vi "Packet1+Packet2.vi"() -> ()   [LabVIEW 2012]
uses:
  <vilib>/addons/Modulation/Digital/General/MT Generate PSK System Parameters(M).vi
  <instrlib>/niUSRP/niUSRP Write Tx Data (CDB Cluster).vi
  <vilib>/addons/Modulation/niDMT.lvlib
panel:
  out "Numeric 2":i32
  in  "Stop the \nTransmission":bool
  out "millisecond timer value 3":u32
  out "Numeric":u32
  out "output cluster":T1
  in  "Referance Cluster":T1={"Tx IQ Sampling\nRate [s/sec]"=500000.0, "Tx Frequency [Hz]"=2500000000.0, "Tx Gain [dB]"=0.0, "Tx Antenna"="TX1"} {"Tx Gain [dB]" format="%#.6p"; "Tx Frequency [Hz]" format="%#.6p"; "Tx IQ Sampling\nRate [s/sec]" format="%#.6p"}
  out "Transmission\n       Stop":bool
  in  "end of data?":bool
  out "Constellation Graph 2":T2(graph) caption="Constellation Graph"
  in  "autoscale 2":bool caption="autoscale"
  out "error out 3":errorcluster
  in  "Tab Control 2":T3(tab)
  in  "Transmitted Message":string
  out "M-ary":i32
  in  "Packet Parameters 2":T4={"Guard Bits "=30, "Sync Bits"=20, "Message Bits"=128}
  in  "Packet Pad \n[samples] 2":i32=200
  in  "Blank Frame \n[samples] 2":i32=500
  out "Number of Packets in Message 2":i32=46
  in  "PN sequence order\nfor Sync Bits 2":i32=31 caption="PN sequence order (9)"
  in  "Packet Repeat 2":i32=2
  in  "Pulse Shaping Filter Parameters 2":T5={"Alpha"=0.5, "Filter Length"=6, "TX Filter"=enum."Root Raised Cos"} caption="Pulse Shaping Filter" {"Alpha" format="%.2f"}
  out "Actual Tx Parameters 2":T1={"Tx IQ Sampling\nRate [s/sec]"=200000.0, "Tx Frequency [Hz]"=2500000000.0, "Tx Gain [dB]"=0.0, "Tx Antenna"="TX1"} {"Tx Gain [dB]" format="%#.6p"; "Tx Frequency [Hz]" format="%#.6p"; "Tx IQ Sampling\nRate [s/sec]" format="%#.6p"}
  out "error out 2":errorcluster
  in  "Queue Length 2":i32=10
  in  "BPSK System Parameters 9":T6={"Samples per Symbol"=8, "symbol map"=[], "Differential PSK"=enum."disable", "PSK type"=0} caption="BPSK System Parameters" {"PSK type" items=["normal", "shifted", "offset"]; "symbol map" format="%.3f"}
  in  "BPSK System Parameters 8":T6={"Samples per Symbol"=8, "symbol map"=[], "Differential PSK"=enum."disable", "PSK type"=0} caption="BPSK System Parameters" {"PSK type" items=["normal", "shifted", "offset"]; "symbol map" format="%.3f"}
  in  "BPSK System Parameters 7":T6={"Samples per Symbol"=8, "symbol map"=[], "Differential PSK"=enum."disable", "PSK type"=0} caption="BPSK System Parameters" {"PSK type" items=["normal", "shifted", "offset"]; "symbol map" format="%.3f"}
  in  "BPSK System Parameters 6":T6={"Samples per Symbol"=8, "symbol map"=[], "Differential PSK"=enum."disable", "PSK type"=0} caption="BPSK System Parameters" {"PSK type" items=["normal", "shifted", "offset"]; "symbol map" format="%.3f"}
  in  "BPSK System Parameters 5":T6={"Samples per Symbol"=8, "symbol map"=[], "Differential PSK"=enum."disable", "PSK type"=0} caption="BPSK System Parameters" {"PSK type" items=["normal", "shifted", "offset"]; "symbol map" format="%.3f"}
  in  "BPSK System Parameters 4":T6={"Samples per Symbol"=8, "symbol map"=[], "Differential PSK"=enum."disable", "PSK type"=0} caption="BPSK System Parameters" {"PSK type" items=["normal", "shifted", "offset"]; "symbol map" format="%.3f"}
  in  "BPSK System Parameters 3":T6={"Samples per Symbol"=8, "symbol map"=[], "Differential PSK"=enum."disable", "PSK type"=0} caption="BPSK System Parameters" {"PSK type" items=["normal", "shifted", "offset"]; "symbol map" format="%.3f"}
  out "Symbol Rate\n[symbols/sec] 2":dbl=25000.0 format="%#.6p"
  out "millisecond timer value":u32
  in  "Tab Control":T3(tab)
  in  "Enter Control Signal\n         (1,2 or 3)":string
  out "The Transmission of \nControl Signal is stopped":bool
  out "Constellation Graph":T2(graph)
  out "Required \nPower Gain":dbl
  in  "Packet Parameters":T4={"Guard Bits "=30, "Sync Bits"=20, "Message Bits"=128}
  in  "Packet Pad \n[samples]":i32=200
  in  "Blank Frame \n[samples]":i32=500
  out "Number of Packets in Message":i32=46
  in  "PN sequence order\nfor Sync Bits":i32=31 caption="PN sequence order (9)"
  in  "Packet Repeat":i32=2
  in  "Select PSK Modulation Format":T7(tab)=enum."QPSK" caption="PSK"
  in  "BPSK System Parameters":T6={"Samples per Symbol"=8, "symbol map"=[], "Differential PSK"=enum."disable", "PSK type"=0} {"PSK type" items=["normal", "shifted", "offset"]; "symbol map" format="%.3f"}
  in  "QPSK System Parameters":T6={"Samples per Symbol"=8, "symbol map"=[], "Differential PSK"=enum."disable", "PSK type"=0} {"PSK type" items=["normal", "shifted", "offset"]; "symbol map" format="%.3f"}
  in  "pi/4 DQPSK System Parameters":T6={"Samples per Symbol"=8, "symbol map"=[], "Differential PSK"=enum."enable", "PSK type"=1} {"PSK type" items=["normal", "shifted", "offset"]; "symbol map" format="%.3f"}
  in  "OQPSK System Parameters":T6={"Samples per Symbol"=8, "symbol map"=[], "Differential PSK"=enum."disable", "PSK type"=2} {"PSK type" items=["normal", "shifted", "offset"]; "symbol map" format="%.3f"}
  in  "8-PSK System Parameters":T6={"Samples per Symbol"=8, "symbol map"=[], "Differential PSK"=enum."disable", "PSK type"=0} {"PSK type" items=["normal", "shifted", "offset"]; "symbol map" format="%.3f"}
  in  "16-PSK System Parameters":T6={"Samples per Symbol"=8, "symbol map"=[], "Differential PSK"=enum."disable", "PSK type"=0} {"PSK type" items=["normal", "shifted", "offset"]; "symbol map" format="%.3f"}
  in  "M":i32=4 min=2 step=2
  in  "Custom System Parameters":T6={"Samples per Symbol"=8, "symbol map"=[], "Differential PSK"=enum."disable", "PSK type"=0} {"PSK type" items=["normal", "shifted", "offset"]; "symbol map" format="%.3f"}
  in  "Pulse Shaping Filter Parameters":T5={"Alpha"=0.5, "Filter Length"=6, "TX Filter"=enum."Root Raised Cos"} caption="Pulse Shaping Filter" {"Alpha" format="%.2f"}
  in  "Tx Parameters":T1={"Tx IQ Sampling\nRate [s/sec]"=500000.0, "Tx Frequency [Hz]"=2500000000.0, "Tx Gain [dB]"=0.0, "Tx Antenna"="TX1"} {"Tx Gain [dB]" format="%#.6p"; "Tx Frequency [Hz]" format="%#.6p"; "Tx IQ Sampling\nRate [s/sec]" format="%#.6p"}
  out "Actual Tx Parameters":T1={"Tx IQ Sampling\nRate [s/sec]"=200000.0, "Tx Frequency [Hz]"=2500000000.0, "Tx Gain [dB]"=0.0, "Tx Antenna"="TX1"} {"Tx Gain [dB]" format="%#.6p"; "Tx Frequency [Hz]" format="%#.6p"; "Tx IQ Sampling\nRate [s/sec]" format="%#.6p"}
  in  "USRP IP address":refnum<k15>="192.168.10.2"
  out "error out":errorcluster
  in  "Queue Length":i32=10
  in  "autoscale":bool
  out "Symbol Rate\n[symbols/sec]":dbl=25000.0 format="%#.6p"
  in  "stop":bool
  # "Guard\nBand"
  # "Sync\nSeq"
  # "Packet\nNumber"
  # "Pad\nData"
  # "Blank\nFrame"
  # "Data"
  # "Guard\nBand"
  # "Sync\nSeq"
  # "Packet\nNumber"
  # "Pad\nData"
  # "Blank\nFrame"
  # "Data"
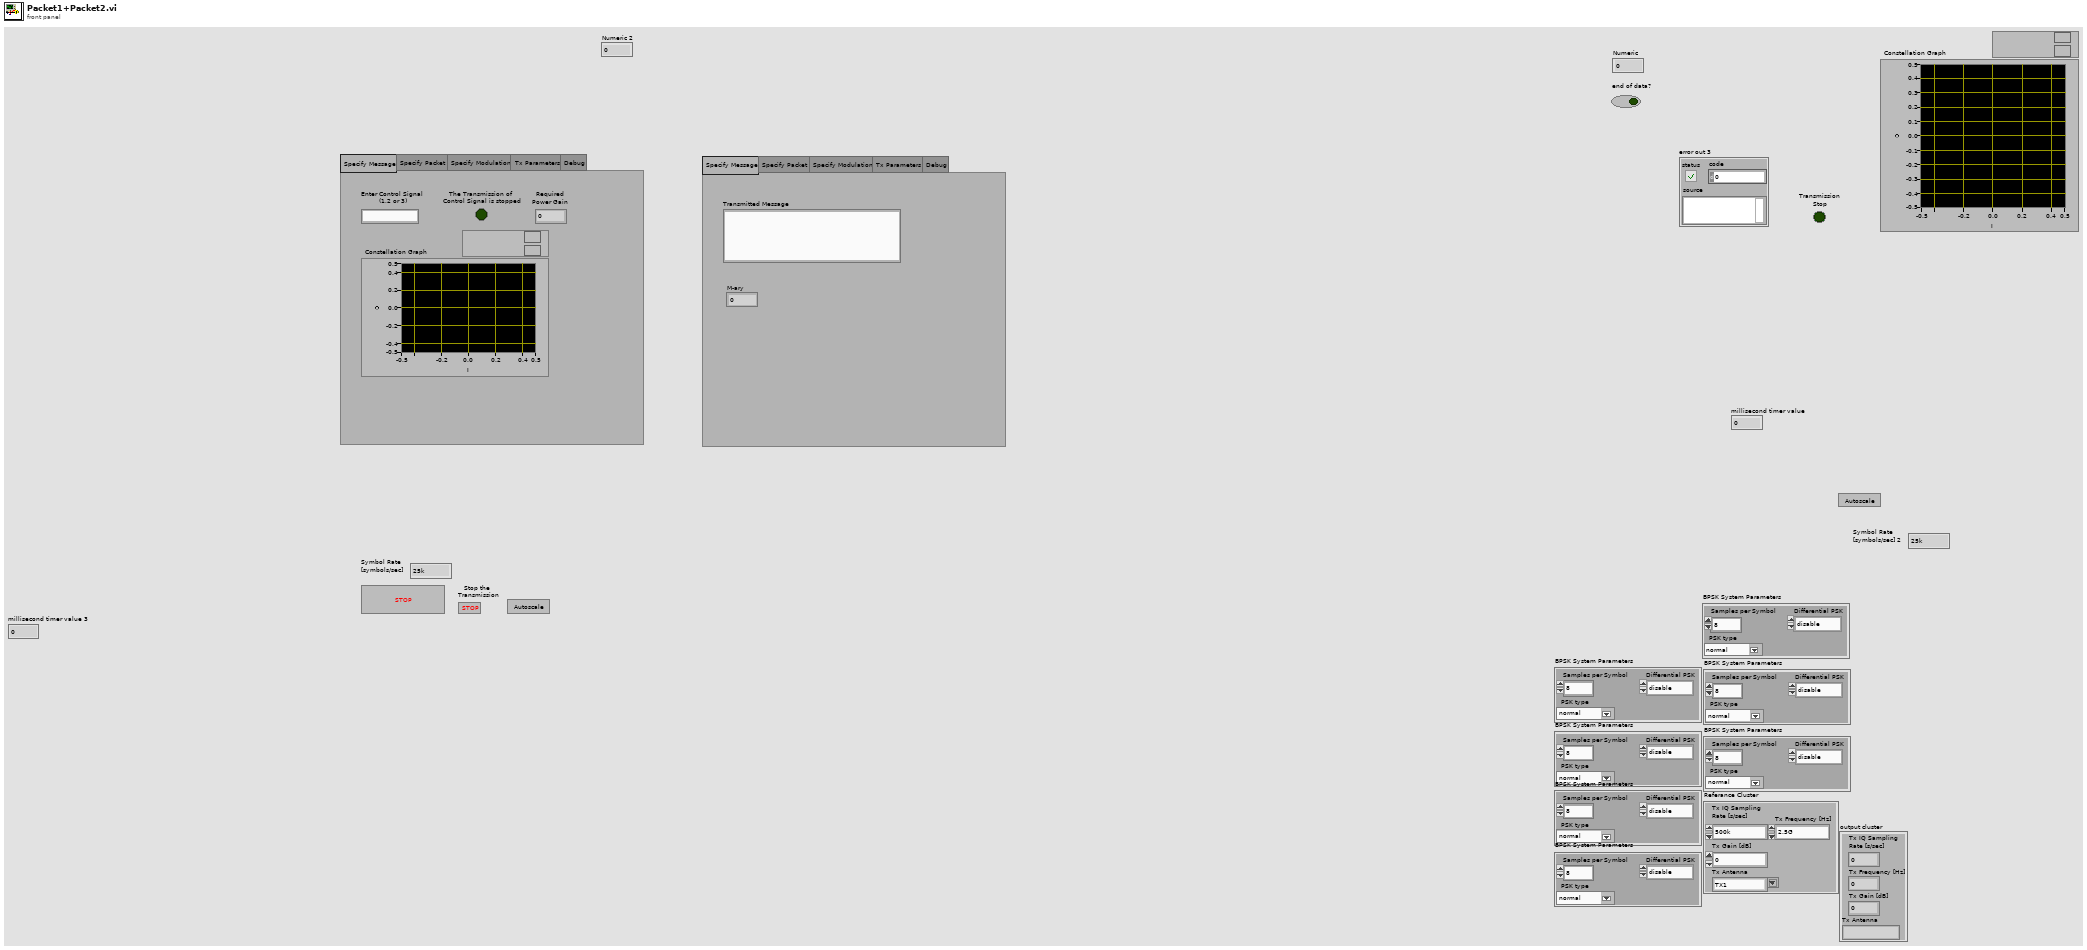
[diagram p1: front panel]
types:
  T1 = cluster{"Tx IQ Sampling\nRate [s/sec]":dbl, "Tx Frequency [Hz]":dbl, "Tx Gain [dB]":dbl, "Tx Antenna":string}
  T2 = cluster{"Decimated Array":dbl[], "Decimated Array":dbl[]}[]
  T3 = enum32{"Specify Message", "Specify Packet", "Specify Modulation", "Tx Parameters", "Debug"}
  T4 = cluster{"Guard Bits ":i32, "Sync Bits":i32, "Message Bits":i32}
  T5 = cluster{"Alpha":dbl, "Filter Length":i32, "TX Filter":enum16{"none", "Raised Cosine", "Root Raised Cos", "Gaussian"}}
  T6 = cluster{"Samples per Symbol":i32, "symbol map":cdb[], "Differential PSK":enum16{"disable", "enable"}, "PSK type":u16}
  T7 = enum32{"BPSK", "QPSK", "pi/4DQPSK", "OQPSK", "8-PSK", "16-PSK", "Custom"}
  T8 = cluster{"samples per symbol (16)":i32, "symbol map":cdb[], "differential PSK":enum16{"disable", "enable"}, "PSK type":u16}
  T9 = cluster{"s? t:f":cluster{"t0":dbl, "dt":dbl, "Y":cdb[]}, i32}
  T10 = cluster{"output complex waveform":cluster{"t0":dbl, "dt":dbl, "Y":cdb[]}, i32}
  T11 = cluster{"constellation":dbl[], "oversampled data":dbl[]}[]
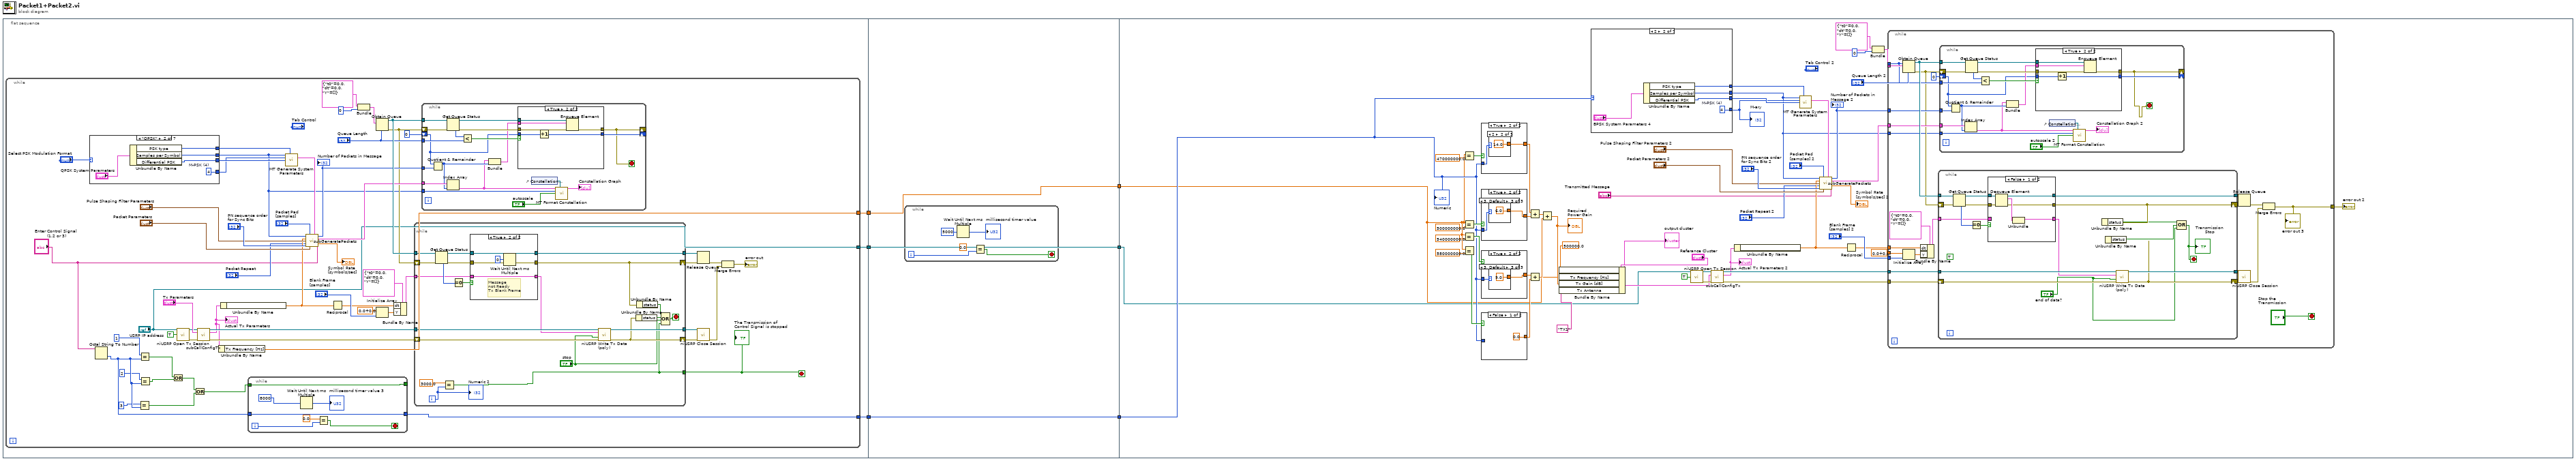
[diagram p0: block diagram]
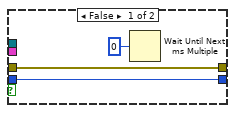
[diagram p2: hidden frame]
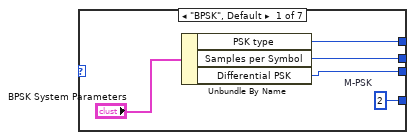
[diagram p3: hidden frame]
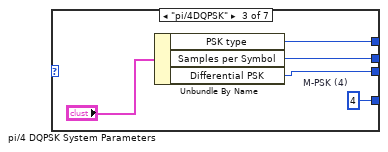
[diagram p4: hidden frame]
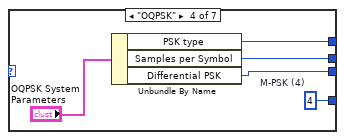
[diagram p5: hidden frame]
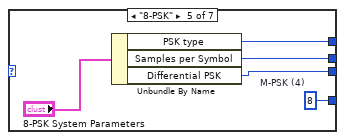
[diagram p6: hidden frame]
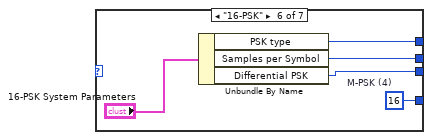
[diagram p7: hidden frame]
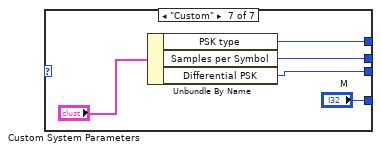
[diagram p8: hidden frame]
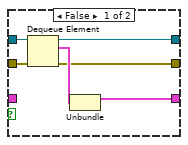
[diagram p9: hidden frame]
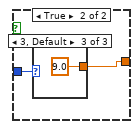
[diagram p10: hidden frame]
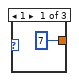
[diagram p11: hidden frame]
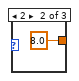
[diagram p12: hidden frame]
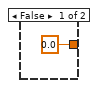
[diagram p13: hidden frame]
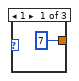
[diagram p14: hidden frame]
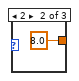
[diagram p15: hidden frame]
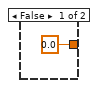
[diagram p16: hidden frame]
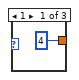
[diagram p17: hidden frame]
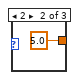
[diagram p18: hidden frame]
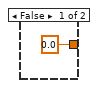
[diagram p19: hidden frame]
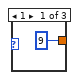
[diagram p20: hidden frame]
diagram:
  n1 = flat-sequence {
    tunnel: [w9] -> w5
    tunnel: [w8] -> w3
    tunnel: [w7] -> w1
    tunnel: [w169] -> w6
    tunnel: w5 -> [w169]
    tunnel: [w168] -> w4
    tunnel: w3 -> [w168]
    tunnel: [w167] -> w2
    tunnel: w1 -> [w167]
    tunnel: w6 -> [w177]
    tunnel: w4 -> [w176]
    tunnel: w2 -> [w175]
    frame #0 {
      n2 = while {
        tunnel: [w15] -> w9
        tunnel: [w13] -> w8
        tunnel: ["USRP IP address"] -> w7
        stop <- w11 stop-if-true
        n3 = case shown="\"QPSK\"" "Select PSK Modulation Format" {
          tunnel: [w102 w106 w114 w119 w124 w130 w133] -> w27
          tunnel: [w103 w108 w113 w118 w123 w129 w134] -> w64
          tunnel: [w105 w110 w115 w120 w122 w128 "M"] -> w46
          tunnel: [w104 w109 w112 w117 w125 w127 w135] -> w35
          frame "BPSK", Default {
            w105 = 2  # M-PSK
            n4 = Unbundle By Name("BPSK System Parameters") -> ("PSK type"=w104:u16, "Samples per Symbol"=w102:i32, "Differential PSK"=w103:enum16{"disable", "enable"})
          }
          frame "QPSK" {
            w110 = 4  # M-PSK (4)
            n5 = Unbundle By Name("QPSK System Parameters") -> ("PSK type"=w109:u16, "Samples per Symbol"=w106:i32, "Differential PSK"=w108:enum16{"disable", "enable"})
          }
          frame "pi/4DQPSK" {
            w115 = 4  # M-PSK (4)
            n6 = Unbundle By Name("pi/4 DQPSK System Parameters") -> ("PSK type"=w112:u16, "Samples per Symbol"=w114:i32, "Differential PSK"=w113:enum16{"disable", "enable"})
          }
          frame "OQPSK" {
            w120 = 4  # M-PSK (4)
            n7 = Unbundle By Name("OQPSK System Parameters") -> ("PSK type"=w117:u16, "Samples per Symbol"=w119:i32, "Differential PSK"=w118:enum16{"disable", "enable"})
          }
          frame "8-PSK" {
            w122 = 8  # M-PSK (4)
            n8 = Unbundle By Name("8-PSK System Parameters") -> ("PSK type"=w125:u16, "Samples per Symbol"=w124:i32, "Differential PSK"=w123:enum16{"disable", "enable"})
          }
          frame "16-PSK" {
            w128 = 16  # M-PSK (4)
            n9 = Unbundle By Name("16-PSK System Parameters") -> ("PSK type"=w127:u16, "Samples per Symbol"=w130:i32, "Differential PSK"=w129:enum16{"disable", "enable"})
          }
          frame "Custom" {
            n10 = Unbundle By Name("Custom System Parameters") -> ("PSK type"=w135:u16, "Samples per Symbol"=w133:i32, "Differential PSK"=w134:enum16{"disable", "enable"})
          }
        }
        n11 = Octal String To Number(4:"Enter Control Signal\n         (1,2 or 3)") -> (0:w19:u32)  [unwired: 2 in, 1 out]
        n12 = Equal?(x=3, y=w19) -> (x = y?=w21:bool)
        n13 = Equal?(x=1, y=w19) -> (x = y?=w24:bool)
        n14 = Equal?(x=2, y=w19) -> (x = y?=w23:bool)
        n15 = Or(x=w24, y=w23) -> (x .or. y?=w22:bool)
        n16 = call <instrlib>:"niUSRP Open Tx Session.vi"("device names"="USRP IP address", "reset"=TRUE) -> ("session handle out"=w38:refnum<k15>, "error out"=w37:errorcluster)  [unwired: 12 in]
        n17 = Or(x=w22, y=w21) -> (x .or. y?=w20:bool)
        n18 = call "subCallConfigTx.vi"("session handle"=w38, "Tx Parameters"="Tx Parameters", "error in"=w37) -> ("session handle out"=w45:refnum<k15>, "Actual Tx Parameters"=w14:T1, "error out"=w50:errorcluster)  [unwired: 10 in]
        "Actual Tx Parameters" <- w14
        n19 = Unbundle By Name(w14) -> ("Tx Frequency [Hz]"=w13:dbl)
        n20 = Unbundle By Name(w14) -> ("Tx IQ Sampling\nRate [s/sec]"=w28:dbl)
        n21 = while {
          tunnel: w20 -> [w71]
          tunnel: [w71] -> _
          tunnel: w19 -> [w70]
          tunnel: [w70] -> w15
          i -> [w68]
          stop <- w67 stop-if-true
          n22 = Wait Until Next ms Multiple(millisecond multiple=u32 8000) -> (millisecond timer value=→"millisecond timer value 3":u32)
          n23 = Equal?(x=0.0, y=w68) -> (x = y?=w67:bool)
        }
        n24 = call-poly <vilib>:"MT Generate System Parameters.vi"("samples per symbol (16)"=w27, "PSK type"=w35, "M-PSK (4)"=w46, "differential PSK"=w64) -> ("PSK system parameters"=w36:T8)  [unwired: 9 in, 2 out]
        n25 = call "subGeneratePackets.vi"("Samples per Symbol"=w27, "Packet Pad \n[samples]"="Packet Pad \n[samples]", "PSK system parameters"=w36, "Tx IQ Sampling\nRate [s/sec]"=w28, "Pulse Shaping Filter Parameters"="Pulse Shaping Filter Parameters", "Packet Repeat"="Packet Repeat", "PN sequence order\nfor Sync Bits"="PN sequence order\nfor Sync Bits", "Packet Parameters"="Packet Parameters", "Message Text"="Enter Control Signal\n         (1,2 or 3)") -> ("Number of Packets"=w44:i32, "Packets"=w52:cluster{"t0":dbl, "dt":dbl, "Y":cdb[]}[], "Symbol Rate"=→"Symbol Rate\n[symbols/sec]":dbl)  [unwired: 4 in]
        "Number of Packets in Message" <- w44
        n26 = Reciprocal(x=w28) -> (1/x=w47:dbl)
        n27 = Bundle("s? t:f"=cluster{"t0":dbl, "dt":dbl, "Y":cdb[]} {"t0"=0.0, "dt"=0.0, "Y"=[]}, 0) -> (w55:T9)  [unwired: 1 in]
        n28 = Obtain Queue(max queue size (-1, unlimited)="Queue Length", element data type=w55) -> (queue out=w61:refnum<queue>, error out=w40:errorcluster)  [unwired: 3 in, 1 out]
        n29 = Initialize Array(cdb 0.0+0.0i ("element"), "Blank Frame \n[samples]") -> (w60:cdb[])
        n30 = Bundle By Name(cluster=cluster{"t0":dbl, "dt":dbl, "Y":cdb[]} {"t0"=0.0, "dt"=0.0, "Y"=[]} ("s? t:f"), "dt"=w47, "Y"=w60) -> (w59:cluster{"t0":dbl, "dt":dbl, "Y":cdb[]})
        n31 = while {
          tunnel: w45 -> [w147]
          shift-right: [w144] -> w49
          shift-left: w50 -> [w148]
          tunnel: w61 -> [w156]
          tunnel: w59 -> [w153]
          tunnel: [w152] -> w58
          tunnel: [w146] -> w48
          shift-right: [w141] -> w57
          shift-left: w40 -> [w149]
          tunnel: [w136] -> w11
          i -> [w137]
          stop <- w143 stop-if-true
          n32 = Get Queue Status(queue=w156, error in (no error)=w149) -> (queue out=w151:refnum<queue>, error out=w150:errorcluster, # elements in queue=w155:i32)  [unwired: 1 in, 5 out]
          n33 = Equal?(x=3000.0, y=w137) -> (x = y?=w136:bool)
          n34 = Equal To 0?(x=w155) -> (x = 0?=w154:bool)
          n35 = case shown="True" w154 {
            tunnel: w153 -> [_ w166]
            tunnel: [w158 w166] -> w139
            tunnel: [w162 w164] -> w152
            tunnel: [w157 w165] -> w141
            tunnel: w151 -> [w161 w164]
            tunnel: w150 -> [w160 w165]
            frame False {
              n36 = Dequeue Element(queue=w161, error in (no error)=w160) -> (queue out=w162:refnum<queue>, element=w159:T9, error out=w157:errorcluster)  [unwired: 1 in, 1 out]
              n37 = Unbundle(w159) -> ("s? t:f"=w158:cluster{"t0":dbl, "dt":dbl, "Y":cdb[]})  [unwired: 1 out]
            }
            frame True {
              # "Message\nnot Ready\nTx Blank Frame"
              n38 = Wait Until Next ms Multiple(millisecond multiple=u32 0) -> ()  [unwired: 1 out]
            }
          }
          n39 = call-poly <instrlib>:"niUSRP Write Tx Data (poly).vi"("session handle"=w147, "data"=w139, "end of data?"="stop", "error in (no error)"=w148) -> ("session handle out"=w146:refnum<k15>, "error out"=w144:errorcluster)  [unwired: 10 in]
          n40 = Unbundle By Name(w144) -> ("status"=w145:bool)
          n41 = Unbundle By Name(w141) -> ("status"=w140:bool)
          n42 = Compound Arithmetic op=OR(w140, w145, "stop", w136) -> (w143:bool)
          "Numeric 2" <- w137
        }
        "The Transmission of \nControl Signal is stopped" <- w11
        n43 = while {
          tunnel: w61 -> [w91]
          shift-right: [w84] -> _
          shift-left: 0 -> [w80]
          tunnel: w52 -> [w81]
          tunnel: "Queue Length" -> [w83]
          tunnel: w44 -> [w82]
          shift-right: [w78] -> _
          shift-left: w40 -> [w86]
          tunnel: w27 -> [w75]
          stop <- w78 stop-if-true
          n44 = Quotient & Remainder(x=w80, y=w82) -> (x-y*floor(x/y)=w79:i32)  [unwired: 1 out]
          n45 = Index Array(array=w81, index=w79) -> (element=w73:cluster{"t0":dbl, "dt":dbl, "Y":cdb[]})
          n46 = Get Queue Status(queue=w91, error in (no error)=w86) -> (queue out=w90:refnum<queue>, error out=w87:errorcluster, # elements in queue=w89:i32)  [unwired: 1 in, 5 out]
          n47 = Less?(x=w89, y=w83) -> (x < y?=w88:bool)
          n48 = Bundle("output complex waveform"=w73, w79) -> (w85:T10)  [unwired: 1 in]
          n49 = case shown="True" w88 {
            tunnel: w87 -> [w92 w100]
            tunnel: w90 -> [_ w99]
            tunnel: [w92 w98] -> w78
            tunnel: w85 -> [_ w97]
            tunnel: w80 -> [w94 w96]
            tunnel: [w94 w95] -> w84
            frame False {
              n50 = Wait Until Next ms Multiple(millisecond multiple=u32 0) -> ()  [unwired: 1 out]
            }
            frame True {
              n51 = Increment(x=w96) -> (x+1=w95:i32)
              n52 = Enqueue Element(queue=w99, element=w97, error in (no error)=w100) -> (error out=w98:errorcluster)  [unwired: 1 in, 2 out]
            }
          }
          n53 = control-ref of="Constellation Graph"() -> (w76:refnum<vi>)
          n54 = call <vilib>:"MT Format Constellation.vi"("waveform"=w73, "constellation reference"=w76, "samples per symbol"=w75, "autoscale"="autoscale") -> ("constellation graph"=→"Constellation Graph":T11)  [unwired: 1 in, 10 out]
        }
        n55 = Release Queue(queue=w58, error in (no error)=w57) -> (error out=w34:errorcluster)  [unwired: 3 out]
        n56 = call <instrlib>:"niUSRP Close Session.vi"("session handle"=w48, "error in (no error)"=w49) -> ("error out"=w33:errorcluster)  [unwired: 13 in]
        n57 = Merge Errors(w34, w33) -> (→"error out":errorcluster)
      }
    }
    frame #1 {
      n58 = while {
        i -> [w172]
        stop <- w171 stop-if-true
        n59 = Wait Until Next ms Multiple(millisecond multiple=u32 5000) -> (millisecond timer value=→"millisecond timer value":u32)
        n60 = Equal?(x=0.0, y=w172) -> (x = y?=w171:bool)
      }
    }
    frame #2 {
      n61 = Equal?(x=w176, y=470000000.0) -> (x = y?=w185:bool)
      n62 = Equal?(x=w176, y=500000000.0) -> (x = y?=w186:bool)
      n63 = Equal?(x=w176, y=540000000.0) -> (x = y?=w187:bool)
      n64 = Equal?(x=w176, y=580000000.0) -> (x = y?=w179:bool)
      n65 = case shown="True" w185 {
        tunnel: [0.0 w245] -> w194
        tunnel: w177 -> [_ w246]
        frame False {
        }
        frame True {
          n66 = case shown="2" w246 {
            tunnel: [9 14.0 18.0] -> w245
            frame 1 {
            }
            frame 2 {
            }
            frame 3, Default {
            }
          }
        }
      }
      n67 = case shown="True" w186 {
        tunnel: [0.0 w239] -> w193
        tunnel: w177 -> [_ w240]
        frame False {
        }
        frame True {
          n68 = case shown="3, Default" w240 {
            tunnel: [4 5.0 6.0] -> w239
            frame 1 {
            }
            frame 2 {
            }
            frame 3, Default {
            }
          }
        }
      }
      n69 = case shown="True" w187 {
        tunnel: [0.0 w233] -> w192
        tunnel: w177 -> [_ w234]
        frame False {
        }
        frame True {
          n70 = case shown="3, Default" w234 {
            tunnel: [7 8.0 9.0] -> w233
            frame 1 {
            }
            frame 2 {
            }
            frame 3, Default {
            }
          }
        }
      }
      n71 = case shown="False" w179 {
        tunnel: [0.0 w227] -> w178
        tunnel: w177 -> [_ w228]
        frame False {
        }
        frame True {
          n72 = case shown="3, Default" w228 {
            tunnel: [7 8.0 9.0] -> w227
            frame 1 {
            }
            frame 2 {
            }
            frame 3, Default {
            }
          }
        }
      }
      n73 = Add(x=w194, y=w193) -> (x+y=w196:dbl)
      n74 = Add(x=w192, y=w178) -> (x+y=w195:dbl)
      n75 = Add(x=w196, y=w195) -> (x+y=w183:dbl)
      "Required \nPower Gain" <- w183
      n76 = Bundle By Name(cluster="Referance Cluster", "Tx IQ Sampling\nRate [s/sec]"=500000.0, "Tx Frequency [Hz]"=w176, "Tx Gain [dB]"=w183, "Tx Antenna"="TX1") -> (w181:T1)
      "output cluster" <- w181
      n77 = case shown="2" w177 {
        tunnel: [w331 w336 w343 w348 w353 w359 w362] -> w200
        tunnel: [w332 w337 w342 w347 w352 w358 w363] -> w225
        tunnel: [w334 w339 w344 w349 w351 w357 0 ("M-PSK (4)")] -> w216
        tunnel: [w333 w338 w341 w346 w354 w356 w364] -> w206
        frame 1 {
          w334 = 2  # M-PSK
          n78 = Unbundle By Name("BPSK System Parameters 3") -> ("PSK type"=w333:u16, "Samples per Symbol"=w331:i32, "Differential PSK"=w332:enum16{"disable", "enable"})
        }
        frame 2 {
          w339 = 4  # M-PSK (4)
          n79 = Unbundle By Name("BPSK System Parameters 4") -> ("PSK type"=w338:u16, "Samples per Symbol"=w336:i32, "Differential PSK"=w337:enum16{"disable", "enable"})
        }
        frame 4 {
          w344 = 4  # M-PSK (4)
          n80 = Unbundle By Name("BPSK System Parameters 5") -> ("PSK type"=w341:u16, "Samples per Symbol"=w343:i32, "Differential PSK"=w342:enum16{"disable", "enable"})
        }
        frame 5 {
          w349 = 4  # M-PSK (4)
          n81 = Unbundle By Name("BPSK System Parameters 6") -> ("PSK type"=w346:u16, "Samples per Symbol"=w348:i32, "Differential PSK"=w347:enum16{"disable", "enable"})
        }
        frame 3, Default {
          w351 = 8  # M-PSK (4)
          n82 = Unbundle By Name("BPSK System Parameters 7") -> ("PSK type"=w354:u16, "Samples per Symbol"=w353:i32, "Differential PSK"=w352:enum16{"disable", "enable"})
        }
        frame 6 {
          w357 = 16  # M-PSK (4)
          n83 = Unbundle By Name("BPSK System Parameters 8") -> ("PSK type"=w356:u16, "Samples per Symbol"=w359:i32, "Differential PSK"=w358:enum16{"disable", "enable"})
        }
        frame 7 {
          n84 = Unbundle By Name("BPSK System Parameters 9") -> ("PSK type"=w364:u16, "Samples per Symbol"=w362:i32, "Differential PSK"=w363:enum16{"disable", "enable"})
        }
      }
      "M-ary" <- w216
      n85 = call <instrlib>:"niUSRP Open Tx Session.vi"("device names"=w175, "reset"=TRUE) -> ("session handle out"=w209:refnum<k15>, "error out"=w208:errorcluster)  [unwired: 12 in]
      n86 = call "subCallConfigTx.vi"("session handle"=w209, "Tx Parameters"=w181, "error in"=w208) -> ("session handle out"=w215:refnum<k15>, "Actual Tx Parameters"=w214:T1, "error out"=w218:errorcluster)  [unwired: 10 in]
      "Actual Tx Parameters 2" <- w214
      n87 = Unbundle By Name(w214) -> ("Tx IQ Sampling\nRate [s/sec]"=w201:dbl)
      n88 = call-poly <vilib>:"MT Generate System Parameters.vi"("samples per symbol (16)"=w200, "PSK type"=w206, "M-PSK (4)"=w216, "differential PSK"=w225) -> ("PSK system parameters"=w207:T8)  [unwired: 9 in, 2 out]
      n89 = call "subGeneratePackets.vi"("Samples per Symbol"=w200, "Packet Pad \n[samples]"="Packet Pad \n[samples] 2", "PSK system parameters"=w207, "Tx IQ Sampling\nRate [s/sec]"=w201, "Pulse Shaping Filter Parameters"="Pulse Shaping Filter Parameters 2", "Packet Repeat"="Packet Repeat 2", "PN sequence order\nfor Sync Bits"="PN sequence order\nfor Sync Bits 2", "Packet Parameters"="Packet Parameters 2", "Message Text"="Transmitted Message") -> ("Number of Packets"=w213:i32, "Packets"=w219:cluster{"t0":dbl, "dt":dbl, "Y":cdb[]}[], "Symbol Rate"=→"Symbol Rate\n[symbols/sec] 2":dbl)  [unwired: 4 in]
      "Number of Packets in Message 2" <- w213
      n90 = Reciprocal(x=w201) -> (1/x=w217:dbl)
      n91 = Bundle("s? t:f"=cluster{"t0":dbl, "dt":dbl, "Y":cdb[]} {"t0"=0.0, "dt"=0.0, "Y"=[]}, 0) -> (w221:T9)  [unwired: 1 in]
      n92 = while {
        tunnel: cdb 0.0+0.0i ("element") -> [w273]
        tunnel: "Blank Frame \n[samples] 2" -> [w272]
        tunnel: w221 -> [w266]
        tunnel: "Queue Length 2" -> [w264]
        tunnel: w219 -> [w263]
        tunnel: w218 -> [w262]
        tunnel: w217 -> [w259]
        tunnel: w215 -> [w258]
        tunnel: w213 -> [w257]
        tunnel: [w252] -> w205
        tunnel: w200 -> [w251]
        stop <- "Stop the \nTransmission" stop-if-true
        n93 = Obtain Queue(max queue size (-1, unlimited)=w264, element data type=w266) -> (queue out=w271:refnum<queue>, error out=w255:errorcluster)  [unwired: 3 in, 1 out]
        n94 = Initialize Array(w273, w272) -> (w270:cdb[])
        n95 = Bundle By Name(cluster=cluster{"t0":dbl, "dt":dbl, "Y":cdb[]} {"t0"=0.0, "dt"=0.0, "Y"=[]} ("s? t:f"), "dt"=w259, "Y"=w270) -> (w269:cluster{"t0":dbl, "dt":dbl, "Y":cdb[]})
        n96 = while {
          tunnel: w258 -> [w310]
          shift-right: [w307] -> w261
          shift-left: w262 -> [w311]
          tunnel: w271 -> [w319]
          tunnel: w269 -> [w316]
          tunnel: [w315] -> w268
          tunnel: [w309] -> w260
          shift-right: [w306] -> w267
          shift-left: w255 -> [w312]
          stop <- w303 stop-if-true
          (unwired) TRUE
          n97 = Get Queue Status(queue=w319, error in (no error)=w312) -> (queue out=w314:refnum<queue>, error out=w313:errorcluster, # elements in queue=w318:i32)  [unwired: 1 in, 5 out]
          n98 = Equal To 0?(x=w318) -> (x = 0?=w317:bool)
          n99 = case shown="False" w317 {
            tunnel: w316 -> [_ w329]
            tunnel: [w321 w329] -> w304
            tunnel: [w325 w327] -> w315
            tunnel: [w320 w328] -> w306
            tunnel: w314 -> [w324 w327]
            tunnel: w313 -> [w323 w328]
            frame False {
              n100 = Dequeue Element(queue=w324, error in (no error)=w323) -> (queue out=w325:refnum<queue>, element=w322:T9, error out=w320:errorcluster)  [unwired: 1 in, 1 out]
              n101 = Unbundle(w322) -> ("s? t:f"=w321:cluster{"t0":dbl, "dt":dbl, "Y":cdb[]})  [unwired: 1 out]
            }
            frame True {
              # "Message\nnot Ready\nTx Blank Frame"
              n102 = Wait Until Next ms Multiple(millisecond multiple=u32 0) -> ()  [unwired: 1 out]
            }
          }
          n103 = Unbundle By Name(w306) -> ("status"=w305:bool)
          n104 = call-poly <instrlib>:"niUSRP Write Tx Data (poly).vi"("session handle"=w310, "data"=w304, "end of data?"="end of data?", "error in (no error)"=w311) -> ("session handle out"=w309:refnum<k15>, "error out"=w307:errorcluster)  [unwired: 10 in]
          n105 = Unbundle By Name(w307) -> ("status"=w308:bool)
          n106 = Compound Arithmetic op=OR(w305, w308, "end of data?") -> (w303:bool)
          "Transmission\n       Stop" <- w303
        }
        n107 = while {
          tunnel: w271 -> [w292]
          shift-right: [w285] -> _
          shift-left: 0 -> [w281]
          tunnel: w263 -> [w282]
          tunnel: w264 -> [w284]
          tunnel: w257 -> [w283]
          shift-right: [w274] -> _
          shift-left: w255 -> [w287]
          tunnel: w251 -> [w277]
          stop <- w274 stop-if-true
          n108 = Quotient & Remainder(x=w281, y=w283) -> (x-y*floor(x/y)=w280:i32)  [unwired: 1 out]
          n109 = Index Array(array=w282, index=w280) -> (element=w275:cluster{"t0":dbl, "dt":dbl, "Y":cdb[]})
          n110 = Get Queue Status(queue=w292, error in (no error)=w287) -> (queue out=w291:refnum<queue>, error out=w288:errorcluster, # elements in queue=w290:i32)  [unwired: 1 in, 5 out]
          n111 = Less?(x=w290, y=w284) -> (x < y?=w289:bool)
          n112 = Bundle("output complex waveform"=w275, w280) -> (w286:T10)  [unwired: 1 in]
          n113 = case shown="True" w289 {
            tunnel: w288 -> [w293 w301]
            tunnel: w291 -> [_ w300]
            tunnel: [w293 w299] -> w274
            tunnel: w286 -> [_ w298]
            tunnel: w281 -> [w295 w297]
            tunnel: [w295 w296] -> w285
            frame False {
              n114 = Wait Until Next ms Multiple(millisecond multiple=u32 0) -> ()  [unwired: 1 out]
            }
            frame True {
              n115 = Increment(x=w297) -> (x+1=w296:i32)
              n116 = Enqueue Element(queue=w300, element=w298, error in (no error)=w301) -> (error out=w299:errorcluster)  [unwired: 1 in, 2 out]
            }
          }
          n117 = control-ref of="Constellation Graph 2"() -> (w278:refnum<vi>)
          n118 = call <vilib>:"MT Format Constellation.vi"("waveform"=w275, "constellation reference"=w278, "samples per symbol"=w277, "autoscale"="autoscale 2") -> ("constellation graph"=→"Constellation Graph 2":T11)  [unwired: 1 in, 10 out]
        }
        n119 = Release Queue(queue=w268, error in (no error)=w267) -> (error out=w254:errorcluster)  [unwired: 3 out]
        n120 = call <instrlib>:"niUSRP Close Session.vi"("session handle"=w260, "error in (no error)"=w261) -> ("error out"=w253:errorcluster)  [unwired: 13 in]
        n121 = Merge Errors(w254, w253) -> (w252:errorcluster)
        "error out 3" <- w252
      }
      "error out 2" <- w205
      "Numeric" <- w177
    }
  }
